vi "(SUBVI) - Motor Control.vi"(8 "NXT/EV3":T1, 10 "Speed":dbl, 11 "Motors":T2=7 items=["Port A", "Port B", "Port C", "Port D"]) -> (0 "NXT/EV3 2":T1)   [LabVIEW 2016, in "testrobot.lvrbt"]
uses:
  testrobot.lvrbt
  <vilib>/NXT/Subs/LVHSConnector.ctl
  <vilib>/NXT/LegoClasses/BrickReference/BrickReference.lvclass
  <vilib>/NXT/Block Support/NXT_OutputPort.ctl
  <vilib>/NXT/NXTIO Xnodes/NXTIONodeSubVIs/NXTMoveMotors.vi
  <vilib>/NXT/NXTIO Xnodes/NXTIOXNode/NXTIO.xnode
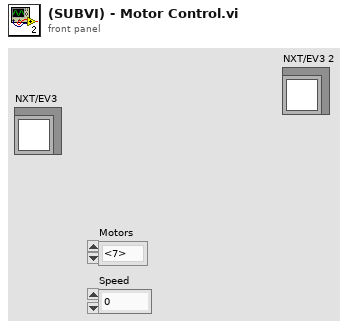
[diagram p1: front panel]
types:
  T1 = typedef "LVHSConnector.ctl" = refnum<class "BrickReference.lvclass">
  T2 = typedef "NXT_OutputPort.ctl" = u8
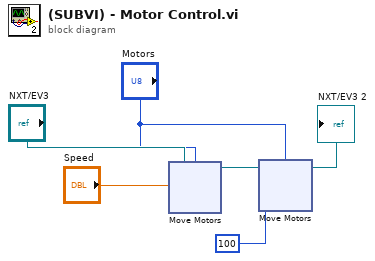
[diagram p0: block diagram]
diagram:
  n1 = xnode "Move Motors"("Power/Speed 1"="Speed", "Motors"="Motors", "NXT/EV3"="NXT/EV3") -> ("NXT/EV3"=w6:T1)
  n2 = xnode "Move Motors"("Power/Speed 1"=100, "Motors"="Motors", "NXT/EV3"=w6) -> ("NXT/EV3"=→"NXT/EV3 2":T1)
